vi "TimingGenerator.vi"(2 "Tick":bool, 3 "Period":u32) -> (0 "TimeSinceLastPulse":u32, 1 "Pulse":bool)   [LabVIEW 2019]
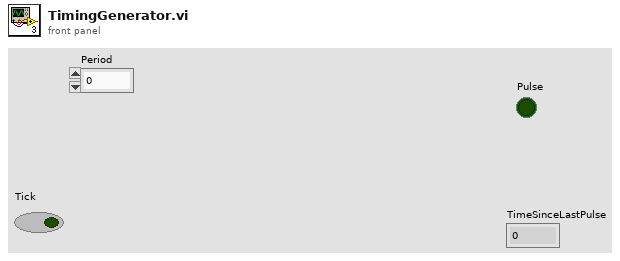
[diagram p1: front panel]
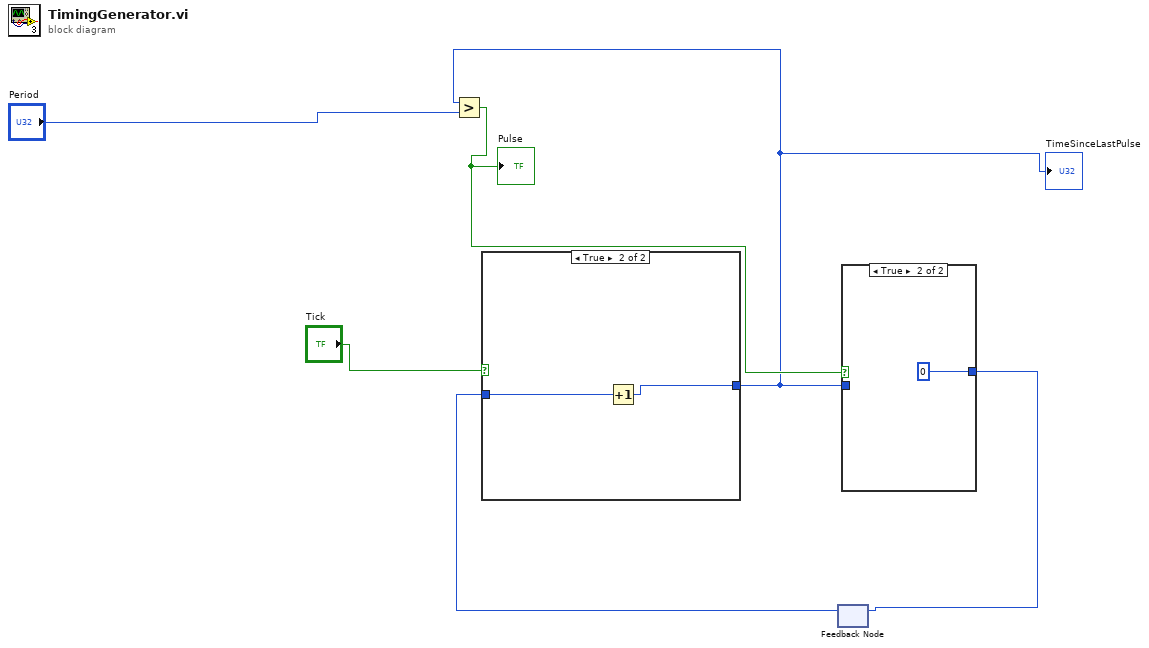
[diagram p0: block diagram]
diagram:
  n1 = feedback #1() -> (w2:u32)  [unwired: 1 in]
  n2 = case shown="True" "Tick" {
    tunnel: [w7 w9] -> w1
    tunnel: w2 -> [w7 w8]
    frame False {
    }
    frame True {
      n3 = Increment(x=w8) -> (x+1=w9:u32)
    }
  }
  "TimeSinceLastPulse" <- w1
  n4 = Greater?(x=w1, y="Period") -> (0:w4:bool)
  "Pulse" <- w4
  n5 = case shown="True" w4 {
    tunnel: [w10 u32 0] -> w3
    tunnel: w1 -> [w10 _]
    frame False {
    }
    frame True {
    }
  }
  n6 = feedback-in #1(w3) -> ()
